vi "extract_calibration_standard_point_locations.vi"(8 "error in (no error)":errorcluster, 9 "Agar (T) Paper (F)":bool, 10 "expected dot radius (camera pixels)":dbl, 11 "Image Src":T1) -> (0 "error out":errorcluster, 2 "Particle Measurements (Pixels)":dbl[][](array[numeric]) format="%.2f", 3 "Image Out (duplicate)":T1)   [LabVIEW 2019]
uses:
  <vilib>/vision/Image Controls.llb/IMAQ Image.ctl
  euclidean_distance_single.vi
  ParametersGlobal.vi
  <vilib>/vision/NI_Vision_Development_Module.lvlib
panel:
  out "Processed Image":T1(plugin-control)
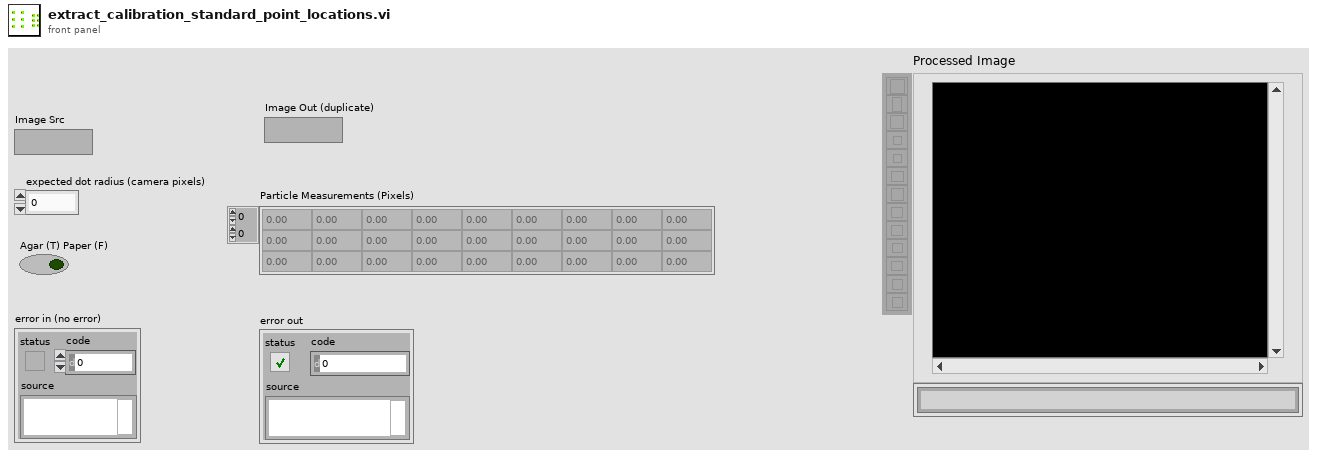
[diagram p1: front panel]
types:
  T1 = typedef "IMAQ Image.ctl" = refnum<image>
  T2 = typedef "Particle Parameters" = i32
  T3 = cluster{"Measurement Parameter":T2, "Range Lower Value":dbl, "Range Upper Value":dbl, "Range":bool, "Measurement Type":bool}
  T4 = typedef "Image Type" = u32
  T5 = cluster{"Measurement Parameter":T2, "Range Lower Value":i32, "Range Upper Value":i32, "Range":bool, "Measurement Type":bool}
  T6 = cluster{"Measurement Parameter":T2, "Range Lower Value":dbl, "Range Upper Value":dbl, "Range":bool, "Measurement Type":bool}[]
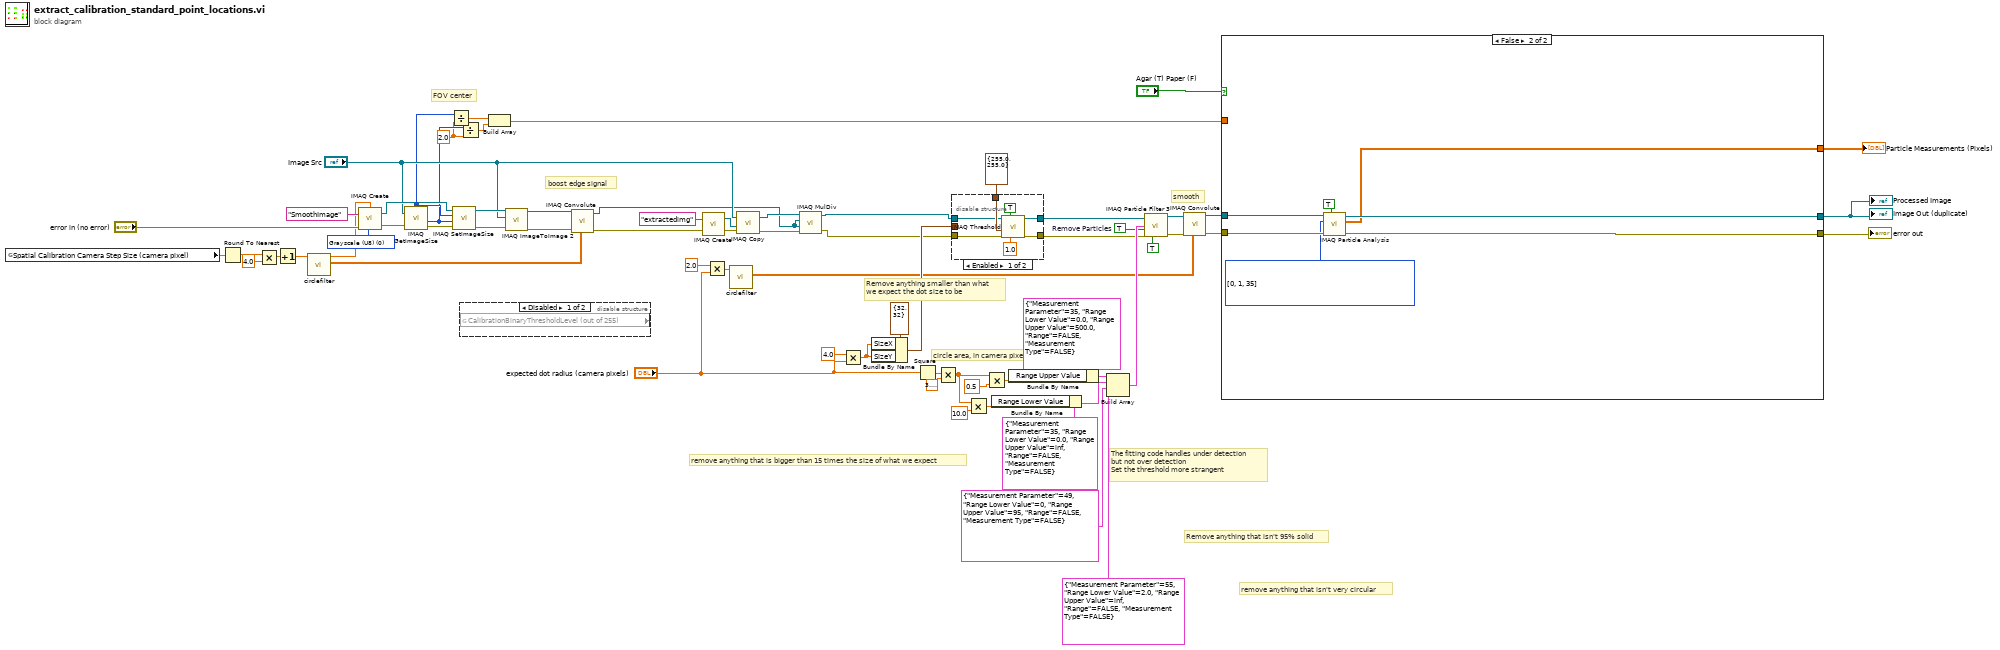
[diagram p0: block diagram]
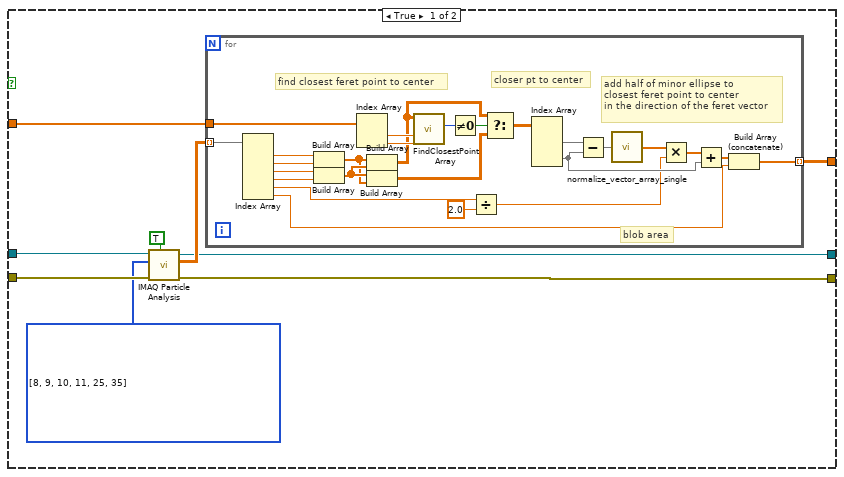
[diagram p2: hidden frame]
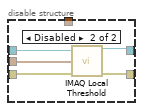
[diagram p4: hidden frame]
diagram:
  w8 = 2.0
  w59 = T4 0 items=["Grayscale (U8)", "Grayscale (I16)", "Grayscale (SGL)", "Complex (CSG)", "RGB (U32)", "HSL (U32)", "RGB (U64)", "Grayscale (U16)"] ("Image Type")
  w61 = TRUE  # Remove Particles
  # "FOV center"
  # "remove anything that isn't very circular"
  # "smooth"
  # "boost edge signal"
  # "remove anything that is bigger than 15 times the size of what we expect"
  # "The fitting code handles under detection\nbut not over detection\nSet the threshold more strangent"
  # "Remove anything that isn't 95% solid"
  # "Remove anything smaller than what\nwe expect the dot size to be"
  # "circle area, in camera pixels squared"
  n1 = global read "ParametersGlobal.vi" "Spatial Calibration Camera Step Size (camera pixel)"() -> (w30:dbl)
  n2 = Round To Nearest(number=w30) -> (nearest integer value=w26:dbl)
  n3 = Multiply(x=w26, y=4.0) -> (x*y=w28:dbl)
  n4 = Increment(x=w28) -> (x+1=w27:dbl)
  n5 = call "circlefilter.vi"("Circle Diameter"=w27) -> ("Filter Weights"=w32:sgl[][], "Image border size"=w31:dbl)  [unwired: 9 in]
  n6 = call "IMAQ Create"("Border Size"=w31, "Image Name"="SmoothImage", "Image Type"=w59, "error in (no error)"="error in (no error)") -> ("New Image"=w57:T1, "error out"=w56:errorcluster)  [unwired: 1 in]
  n7 = call "IMAQ GetImageSize"("Image"="Image Src", "error in (no error)"=w56) -> ("Y Resolution"=w9:i32, "X Resolution"=w10:i32, "error out"=w58:errorcluster)  [unwired: 2 in]
  n8 = Divide(x=w10, y=w8) -> (x/y=w7:dbl)
  n9 = call "IMAQ SetImageSize"("error in (no error)"=w58, "Y Resolution"=w9, "X Resolution"=w10, "Image"=w57) -> ("error out"=w54:errorcluster, "Image Out"=w55:T1)  [unwired: 1 in]
  n10 = Divide(x=w9, y=w8) -> (x/y=w6:dbl)
  n11 = disable-structure shown="Disabled" {
    frame Disabled {
      n12 = global read "ParametersGlobal.vi" "CalibrationBinaryThresholdLevel (out of 255)"() -> ()  [unwired: 1 out]
    }
    frame Enabled {
    }
  }
  n13 = Build Array(w7, w6) -> (w5:dbl[])
  n14 = call "IMAQ ImageToImage 2"("error in (no error)"=w54, "Image Src (Small)"="Image Src", "Image Src (Large)"=w55) -> ("error out"=w37:errorcluster, "Image Dst Out"=w36:T1)  [unwired: 7 in]
  n15 = call "IMAQ Convolute"("Kernel"=w32, "error in (no error)"=w37, "Image Src"=w36) -> ("error out"=w34:errorcluster, "Image Dst Out"=w17:T1)  [unwired: 7 in]
  n16 = call "IMAQ Create"("Image Name"="extractedimg", "error in (no error)"=w34) -> ("New Image"=w33:T1, "error out"=w35:errorcluster)  [unwired: 3 in]
  n17 = Multiply(x=2.0, y="expected dot radius (camera pixels)") -> (x*y=w11:dbl)
  n18 = call "circlefilter.vi"("Circle Diameter"=w11) -> ("Filter Weights"=w14:sgl[][])  [unwired: 9 in, 1 out]
  n19 = call "IMAQ Copy"("error in (no error)"=w35, "Image Dst"=w33, "Image Src"="Image Src") -> ("error out"=w25:errorcluster, "Image Dst Out"=w18:T1)  [unwired: 3 in]
  n20 = call "IMAQ MulDiv"("Image Src A"=w18, "Image Dst"=w17, "Image Src B"=w17, "error in (no error)"=w25) -> ("Image Dst Out"=w23:T1, "error out"=w24:errorcluster)  [unwired: 3 in]
  n21 = Multiply(x=4.0, y="expected dot radius (camera pixels)") -> (x*y=w43:dbl)
  n22 = Bundle By Name(cluster=cluster{"SizeX":i32, "SizeY":i32} {"SizeX"=32, "SizeY"=32} ("Window Size (32x32)"), "SizeX"=w43, "SizeY"=w43) -> (w45:cluster{"SizeX":i32, "SizeY":i32})
  n23 = Square(x="expected dot radius (camera pixels)") -> (x^2=w68:dbl)
  n24 = Multiply(x=w68, y=3.141592653589793) -> (x*y=w50:dbl)
  n25 = disable-structure shown="Enabled" {
    disable-tunnel: w24 -> [w75 w80]
    disable-tunnel: cluster{"Lower value":sgl, "Upper value":sgl} {"Lower value"=255.0, "Upper value"=255.0} ("Range") -> [w74 _]
    disable-tunnel: [w71 w78] -> w22
    disable-tunnel: [w70 w79] -> w62
    disable-tunnel: w23 -> [w69 w77]
    disable-tunnel: w45 -> [_ w76]
    frame Enabled {
      n26 = call "IMAQ Threshold"("Replace Value"=sgl 1.0, "Keep/Replace Value (Replace)"=TRUE, "error in (no error)"=w75, "Range"=w74, "Image Src"=w69) -> ("error out"=w70:errorcluster, "Image Dst Out"=w71:T1)  [unwired: 5 in]
    }
    frame Disabled {
      n27 = call "IMAQ Local Threshold"("Image Src"=w77, "Window Size (32x32)"=w76, "error in (no error)"=w80) -> ("Image Dst Out"=w78:T1, "error out"=w79:errorcluster)  [unwired: 11 in]
    }
  }
  n28 = Multiply(x=w50, y=10.0) -> (x*y=w48:dbl)
  n29 = Multiply(x=w50, y=0.5) -> (x*y=w64:dbl)
  n30 = Bundle By Name(cluster=T3 {"Measurement Parameter"=35, "Range Lower Value"=0.0, "Range Upper Value"=inf, "Range"=FALSE, "Measurement Type"=FALSE} ("Selection Value"), "Range Lower Value"=w48) -> (w47:T3)
  n31 = Bundle By Name(cluster=T3 {"Measurement Parameter"=35, "Range Lower Value"=0.0, "Range Upper Value"=500.0, "Range"=FALSE, "Measurement Type"=FALSE} ("Selection Value"), "Range Upper Value"=w64) -> (w52:T3)
  n32 = Build Array(w52, w47, T5 {"Measurement Parameter"=49, "Range Lower Value"=0, "Range Upper Value"=95, "Range"=FALSE, "Measurement Type"=FALSE} ("Selection Value"), T3 {"Measurement Parameter"=55, "Range Lower Value"=2.0, "Range Upper Value"=inf, "Range"=FALSE, "Measurement Type"=FALSE} ("element")) -> (w66:T6)
  n33 = call "IMAQ Particle Filter 3"("Image Src"=w22, "Selection Values"=w66, "Keep/Remove Particles (F)"=w61, "error in (no error)"=w62, "Reject Border? (F)"=TRUE) -> ("Image Dst Out"=w19:T1, "error out"=w20:errorcluster)  [unwired: 4 in, 5 out]
  n34 = call "IMAQ Convolute"("Kernel"=w14, "error in (no error)"=w20, "Image Src"=w19) -> ("error out"=w15:errorcluster, "Image Dst Out"=w16:T1)  [unwired: 7 in]
  n35 = case shown="False" "Agar (T) Paper (F)" {
    tunnel: w16 -> [w88 w121]
    tunnel: w15 -> [w87 w120]
    tunnel: w5 -> [w85 _]
    tunnel: [w84 w117] -> w4
    tunnel: [w83 w119] -> w3
    tunnel: [w81 w118] -> w2
    frame True {
      w82 = T2[] [8, 9, 10, 11, 25, 35] items=["Center of Mass X", "Center of Mass Y", "First Pixel X", "First Pixel Y", "Bounding Rect Left", "Bounding Rect Top", "Bounding Rect Right", "Bounding Rect Bottom", "Max Feret Diameter Start X", "Max Feret Diameter Start Y", "Max Feret Diameter End X", "Max Feret Diameter End Y", "Max Horiz. Segment Length Left", "Max Horiz. Segment Length Right", "Max Horiz. Segment Length Row", "-", "Bounding Rect Width", "Bounding Rect Height", "Bounding Rect Diagonal", "Perimeter", "Convex Hull Perimeter", "Holes' Perimeter", "Max Feret Diameter", "Equivalent Ellipse Major Axis", "Equivalent Ellipse Minor Axis", "Equivalent Ellipse Minor Axis (Feret)", "Equivalent Rect Long Side", "Equivalent Rect Short Side", "Equivalent Rect Diagonal", "Equivalent Rect Short Side (Feret)", "Average Horiz. Segment Length", "Average Vert. Segment Length", "Hydraulic Radius", "Waddel Disk Diameter", "-", "Area", "Holes' Area", "Particle & Holes' Area", "Convex Hull Area", "Image Area", "-", "Number of Holes", "Number of Horiz. Segments", "Number of Vert. Segments", "-", "Orientation", "Max Feret Diameter Orientation", "-", "% Area/Image Area", "% Area/(Particle & Holes' Area)", "Ratio of Equivalent Ellipse Axes", "Ratio of Equivalent Rect Sides", "-", "Elongation Factor", "Compactness Factor", "Heywood Circularity Factor", "Type Factor", "-", "Sum X", "Sum Y", "Sum XX", "Sum XY", "Sum YY", "Sum XXX", "Sum XXY", "Sum XYY", "Sum YYY", "-", "Moment of Inertia XX", "Moment of Inertia XY", "Moment of Inertia YY", "Moment of Inertia XXX", "Moment of Inertia XXY", "Moment of Inertia XYY", "Moment of Inertia YYY", "Norm. Moment of Inertia XX", "Norm. Moment of Inertia XY", "Norm. Moment of Inertia YY", "Norm. Moment of Inertia XXX", "Norm. Moment of Inertia XXY", "Norm. Moment of Inertia XYY", "Norm. Moment of Inertia YYY", "Hu Moment 1", "Hu Moment 2", "Hu Moment 3", "Hu Moment 4", "Hu Moment 5", "Hu Moment 6", "Hu Moment 7"] ("Pixel Measurements")
      n36 = call "IMAQ Particle Analysis"("Connectivity 4/8 (8)"=TRUE, "error in (no error)"=w87, "Pixel Measurements"=w82, "Image"=w88) -> ("error out"=w83:errorcluster, "Particle Measurements (Pixels)"=w86:dbl[][], "Image Out (duplicate)"=w81:T1)  [unwired: 2 in, 3 out]
      n37 = for {
        tunnel: w86 -> [w96] mode=indexing
        tunnel: w85 -> [w111]
        tunnel: [w90] -> w84 mode=indexing
        # "blob area"
        # "add half of minor ellipse to \nclosest feret point to center\nin the direction of the feret vector"
        # "closer pt to center"
        # "find closest feret point to center"
        n38 = Index Array(array=w96) -> (element #1=w115:dbl, element #2=w114:dbl, element #3=w113:dbl, element #4=w112:dbl, element #5=w95:dbl, element #6=w91:dbl)  [unwired: 6 in]
        n39 = Build Array(w115, w114) -> (w104:dbl[])
        n40 = Build Array(w113, w112) -> (w105:dbl[])
        n41 = Index Array(array=w111) -> (element #1=w110:dbl, element #2=w109:dbl)  [unwired: 2 in]
        n42 = Build Array(w104, w105) -> (w106:dbl[][])
        n43 = Build Array(w105, w104) -> (w103:dbl[][])
        n44 = call "FindClosestPointArray.vi"("Y"=w109, "X"=w110, "Particle Measurements (Pixels)"=w106) -> ("ShortestDistanceIndex"=w108:i32)  [unwired: 7 in, 1 out]
        n45 = Not Equal To 0?(x=w108) -> (x != 0?=w107:bool)
        n46 = Divide(x=w95, y=2.0) -> (x/y=w93:dbl)
        n47 = Select(t=w106, s=w107, f=w103) -> (s? t:f=w102:dbl[][])
        n48 = Index Array(array=w102) -> (element #1=w101:dbl[], element #2=w97:dbl[])  [unwired: 4 in]
        n49 = Subtract(x=w101, y=w97) -> (x-y=w100:dbl[])
        n50 = call "normalize_vector_array_single.vi"("2 element vector"=w100) -> ("normalized vector out"=w99:sgl[])
        n51 = Multiply(x=w99, y=w93) -> (x*y=w98:dbl[])
        n52 = Add(x=w98, y=w97) -> (x+y=w92:dbl[])
        n53 = Build Array (concatenate)(w92, w91) -> (w90:dbl[])
      }
    }
    frame False {
      w116 = T2[] [0, 1, 35] items=["Center of Mass X", "Center of Mass Y", "First Pixel X", "First Pixel Y", "Bounding Rect Left", "Bounding Rect Top", "Bounding Rect Right", "Bounding Rect Bottom", "Max Feret Diameter Start X", "Max Feret Diameter Start Y", "Max Feret Diameter End X", "Max Feret Diameter End Y", "Max Horiz. Segment Length Left", "Max Horiz. Segment Length Right", "Max Horiz. Segment Length Row", "-", "Bounding Rect Width", "Bounding Rect Height", "Bounding Rect Diagonal", "Perimeter", "Convex Hull Perimeter", "Holes' Perimeter", "Max Feret Diameter", "Equivalent Ellipse Major Axis", "Equivalent Ellipse Minor Axis", "Equivalent Ellipse Minor Axis (Feret)", "Equivalent Rect Long Side", "Equivalent Rect Short Side", "Equivalent Rect Diagonal", "Equivalent Rect Short Side (Feret)", "Average Horiz. Segment Length", "Average Vert. Segment Length", "Hydraulic Radius", "Waddel Disk Diameter", "-", "Area", "Holes' Area", "Particle & Holes' Area", "Convex Hull Area", "Image Area", "-", "Number of Holes", "Number of Horiz. Segments", "Number of Vert. Segments", "-", "Orientation", "Max Feret Diameter Orientation", "-", "% Area/Image Area", "% Area/(Particle & Holes' Area)", "Ratio of Equivalent Ellipse Axes", "Ratio of Equivalent Rect Sides", "-", "Elongation Factor", "Compactness Factor", "Heywood Circularity Factor", "Type Factor", "-", "Sum X", "Sum Y", "Sum XX", "Sum XY", "Sum YY", "Sum XXX", "Sum XXY", "Sum XYY", "Sum YYY", "-", "Moment of Inertia XX", "Moment of Inertia XY", "Moment of Inertia YY", "Moment of Inertia XXX", "Moment of Inertia XXY", "Moment of Inertia XYY", "Moment of Inertia YYY", "Norm. Moment of Inertia XX", "Norm. Moment of Inertia XY", "Norm. Moment of Inertia YY", "Norm. Moment of Inertia XXX", "Norm. Moment of Inertia XXY", "Norm. Moment of Inertia XYY", "Norm. Moment of Inertia YYY", "Hu Moment 1", "Hu Moment 2", "Hu Moment 3", "Hu Moment 4", "Hu Moment 5", "Hu Moment 6", "Hu Moment 7"] ("Real-World Measurements")
      n54 = call "IMAQ Particle Analysis"("Connectivity 4/8 (8)"=TRUE, "error in (no error)"=w120, "Pixel Measurements"=w116, "Image"=w121) -> ("error out"=w119:errorcluster, "Particle Measurements (Pixels)"=w117:dbl[][], "Image Out (duplicate)"=w118:T1)  [unwired: 2 in, 3 out]
    }
  }
  "error out" <- w3
  "Particle Measurements (Pixels)" <- w4
  "Image Out (duplicate)" <- w2
  "Processed Image" <- w2
